vi "BubbleSort.vi"(11 "InputArray":T1[](array[typedef])) -> (3 "SortedArray":T1[](array[typedef]))   [LabVIEW 2016]
uses:
  SSL Detection Ball w ID.ctl
  <vilib>/Analysis/Matrix/Datatypes/RealMatrix.ctl
  <vilib>/Analysis/Matrix/NI_Matrix.lvlib
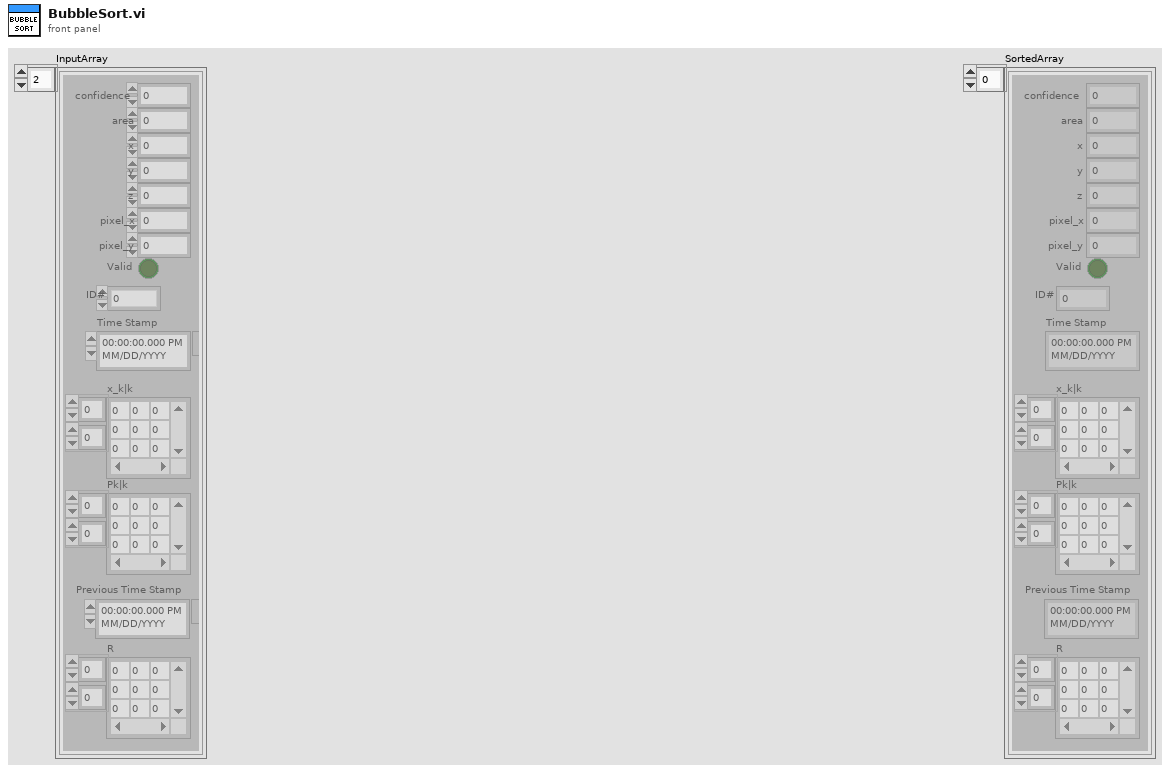
[diagram p1: front panel]
types:
  T1 = typedef "SSL Detection Ball w ID.ctl" = cluster{"x":sgl, "area":u32, "confidence":sgl, "y":sgl, "z":sgl, "pixel_x":sgl, "pixel_y":sgl, "Valid":bool, "Time Stamp":timestamp, "x_k|k":T2, "Pk|k":T2, "ID#":u32, "Previous Time Stamp":timestamp, "R":T2}
  T2 = typedef "NI_Matrix.lvlib/RealMatrix.ctl" = dbl[][]
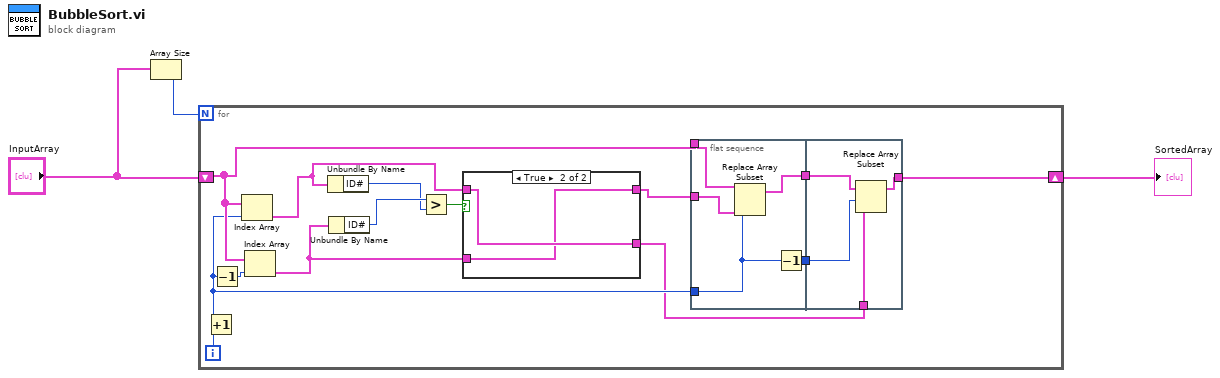
[diagram p0: block diagram]
diagram:
  n1 = Array Size(array="InputArray") -> (size(s)=w2:i32)
  n2 = for {
    N: w2 -> [_]
    shift-right: [w4] -> w1
    shift-left: "InputArray" -> [w10]
    i -> [w9]
    n3 = Increment(x=w9) -> (x+1=w8:i32)
    n4 = Decrement(x=w8) -> (x-1=w13:i32)
    n5 = Index Array(array=w10, index=w8) -> (element=w14:T1)
    n6 = Index Array(array=w10, index=w13) -> (element=w12:T1)
    n7 = Unbundle By Name(w14) -> ("ID#"=w16:u32)
    n8 = Unbundle By Name(w12) -> ("ID#"=w17:u32)
    n9 = Greater?(x=w17, y=w16) -> (0:w15:bool)
    n10 = case shown="True" w15 {
      tunnel: w14 -> [w28 w30]
      tunnel: w12 -> [w27 w29]
      tunnel: [w28 w29] -> w11
      tunnel: [w27 w30] -> w5
      frame False {
      }
      frame True {
      }
    }
    n11 = flat-sequence {
      tunnel: w11 -> [w21]
      tunnel: w10 -> [w20]
      tunnel: w8 -> [w19]
      tunnel: [w22] -> w7
      tunnel: [w18] -> w6
      tunnel: w7 -> [w25]
      tunnel: w6 -> [w26]
      tunnel: w5 -> [w24]
      tunnel: [w23] -> w4
      frame #0 {
        n12 = Replace Array Subset(array=w20, new element=w21, index=w19) -> (w18:T1[])
        n13 = Decrement(x=w19) -> (x-1=w22:i32)
      }
      frame #1 {
        n14 = Replace Array Subset(array=w26, new element=w24, index=w25) -> (w23:T1[])
      }
    }
  }
  "SortedArray" <- w1
